vi "TimeChannelStorage.vi"(2 "error in (no error)":errorcluster, 3 "Timing Channel Settings":T1[][](array[typedef]) {"FrontPanelTime" format="%.3p"; "Pulse width (s)" format="%.3p"; "Delay (s)" format="%.3p"}, 4 "Data Value Reference in":refnum<data-value>) -> (0 "error out":errorcluster)   [LabVIEW 2013]
uses:
  <vilib>/MDSplus/Classes/Tree_Class/Tree.lvclass
  Controls/TimingChannelSettings.ctl
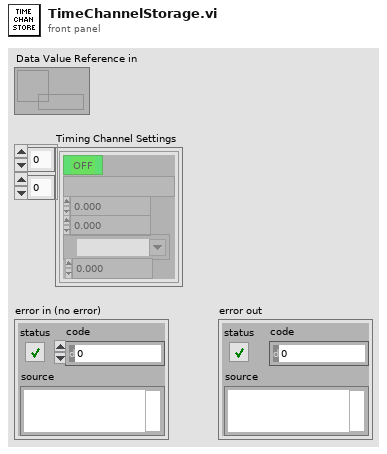
[diagram p1: front panel]
types:
  T1 = typedef "TimingChannelSettings.ctl" = cluster{"Delay (s)":dbl, "Pulse width (s)":dbl, "Active":bool, "Channel Name":string, "counter":tag, "FrontPanelTime":dbl}
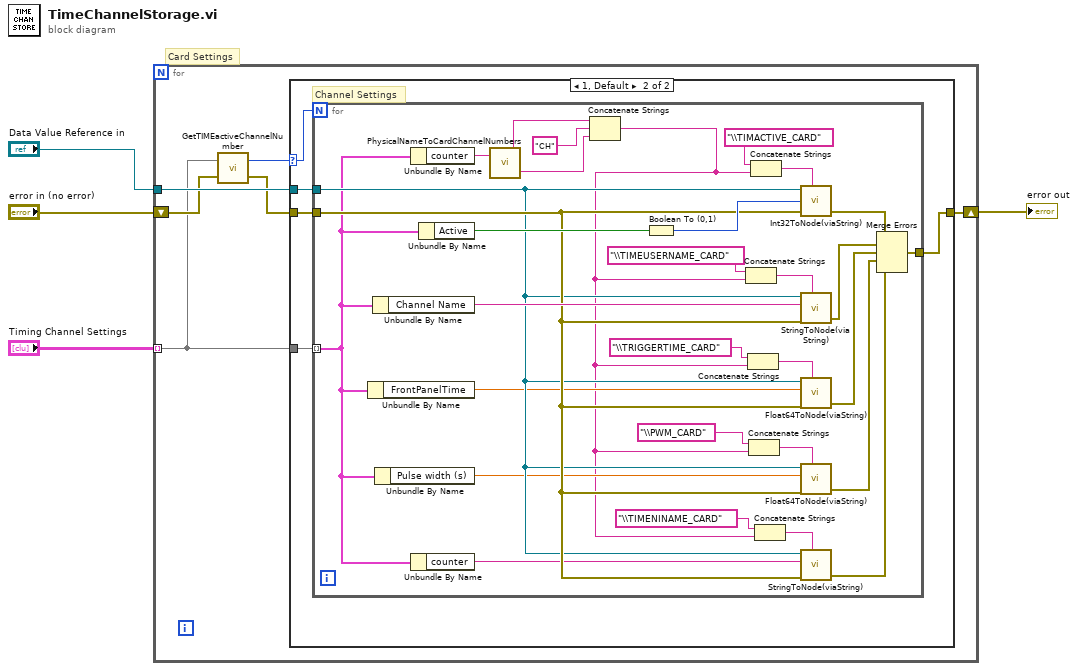
[diagram p0: block diagram]
diagram:
  # "Card Settings"
  n1 = for {
    shift-right: [w9] -> w1
    shift-left: "error in (no error)" -> [w8]
    tunnel: "Timing Channel Settings" -> [w6] mode=indexing
    tunnel: "Data Value Reference in" -> [w10]
    n2 = call "GetTIMEactiveChannelNumber.vi"("error in (no error)"=w8, "Timing Channel Settings"=w6) -> ("error out"=w7:errorcluster, "Numeric"=w5:i16)
    n3 = case shown="1, Default" w5 {
      selector: w5 -> [_ w12]
      tunnel: w10 -> [_ w16]
      tunnel: [w11 w15] -> w9
      tunnel: w6 -> [_ w14]
      tunnel: w7 -> [w11 w13]
      frame 0 {
      }
      frame 1, Default {
        # "Channel Settings"
        n4 = for {
          N: w12 -> [_]
          tunnel: w13 -> [w37]
          tunnel: w14 -> [w26] mode=indexing
          tunnel: w16 -> [w36]
          tunnel: [w27] -> w15
          n5 = Unbundle By Name(w26) -> ("FrontPanelTime"=w33:dbl)
          n6 = Unbundle By Name(w26) -> ("Channel Name"=w41:string)
          n7 = Unbundle By Name(w26) -> ("Pulse width (s)"=w34:dbl)
          n8 = Unbundle By Name(w26) -> ("counter"=w25:tag)
          n9 = Unbundle By Name(w26) -> ("counter"=w35:tag)
          n10 = Unbundle By Name(w26) -> ("Active"=w43:bool)
          n11 = call "PhysicalNameToCardChannelNumbers.vi"("NI Physical Channel"=w25) -> ("Channel #"=w23:string, "Card #"=w24:string)  [unwired: 1 in]
          n12 = Concatenate Strings(w24, "CH" ("string"), w23) -> (w18:string)
          n13 = Boolean To (0,1)(Boolean=w43) -> (0, 1=w45:i16)
          n14 = Concatenate Strings("\\TIMEUSERNAME_CARD" ("string"), w18) -> (w42:string)
          n15 = Concatenate Strings("\\TRIGGERTIME_CARD" ("string"), w18) -> (w40:string)
          n16 = Concatenate Strings("\\PWM_CARD" ("string"), w18) -> (w39:string)
          n17 = Concatenate Strings("\\TIMACTIVE_CARD" ("string"), w18) -> (w44:string)
          n18 = Concatenate Strings("\\TIMENINAME_CARD" ("string"), w18) -> (w38:string)
          n19 = call "Int32ToNode(viaString).vi"("Tree DVR in"=w36, "I32 in"=w45, "error in (no error)"=w37, "NodePath"=w44) -> ("error out"=w32:errorcluster)  [unwired: 1 in, 2 out]
          n20 = call "StringToNode(viaString).vi"("Tree DVR in"=w36, "String value in"=w41, "error in (no error)"=w37, "NodePath"=w42) -> ("error out"=w31:errorcluster)  [unwired: 1 in, 2 out]
          n21 = call "Float64ToNode(viaString).vi"("Tree DVR in"=w36, "DBL in"=w33, "error in"=w37, "NodePath"=w40) -> ("error out"=w30:errorcluster)  [unwired: 1 in, 2 out]
          n22 = call "Float64ToNode(viaString).vi"("Tree DVR in"=w36, "DBL in"=w34, "error in"=w37, "NodePath"=w39) -> ("error out"=w29:errorcluster)  [unwired: 1 in, 2 out]
          n23 = call "StringToNode(viaString).vi"("Tree DVR in"=w36, "String value in"=w35, "error in (no error)"=w37, "NodePath"=w38) -> ("error out"=w28:errorcluster)  [unwired: 1 in, 2 out]
          n24 = Merge Errors(w32, w31, w30, w29, w28) -> (w27:errorcluster)
        }
      }
    }
  }
  "error out" <- w1
